vi "testAndMeasure.vi"() -> ()   [LabVIEW 2016]
uses:
  Anemometry/Anemometry Sub Vis/Controls/Post_Process.ctl
  Anemometry/Anemometry Sub Vis/Controls/Save_Data.ctl
  Anemometry/Anemometry Sub Vis/Controls/Setup.ctl
  Anemometry/Anemometry Sub Vis/Globals/Meas_global.vi
panel:
  in  "Measure (seconds)":dbl=10.0
  in  "Stop Button":bool
  in  "ResultsFilename":string="StaircaseTest"
  in  "settling(s)":u32=10
  out "conc":dbl=2.0 format="%.2f"
  out "flow":dbl=10.0 format="%.2f"
  in  "flowStep":dbl=10.0
  in  "flowMax":dbl=100.0
  in  "concMax":dbl=10.0
  in  "concStep":dbl=1.0
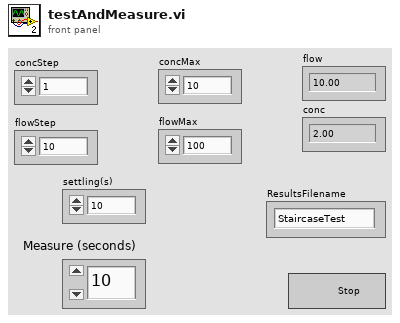
[diagram p1: front panel]
types:
  T1 = typedef "Setup.ctl" = enum16{"Run Program", "Show Setup", "Save Current Setup", "Setup Front Panel"}
  T2 = typedef "Save_Data.ctl" = enum16{"Save No Data", "Save Data"}
  T3 = typedef "Post_Process.ctl" = enum16{"Take New Data", "Post Process Raw Data File"}
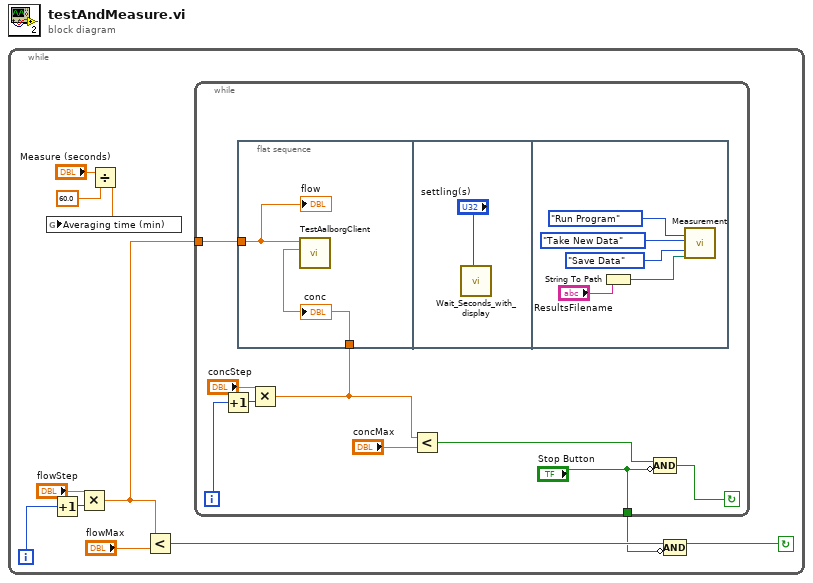
[diagram p0: block diagram]
diagram:
  n1 = while {
    i -> [w9]
    stop <- w2 continue-if-true
    n2 = Increment(x=w9) -> (x+1=w10:i32)
    n3 = Multiply(x="flowStep", y=w10) -> (x*y=w6:dbl)
    n4 = Divide(x="Measure (seconds)", y=60.0 ("x")) -> (x/y=w3:dbl)
    n5 = global write "Meas_global.vi" "Averaging time (min)"(w3) -> ()
    n6 = Less?(x=w6, y="flowMax") -> (x < y?=w8:bool)
    n7 = while {
      tunnel: w6 -> [w16]
      tunnel: ["Stop Button"] -> w1
      i -> [w20]
      stop <- w13 continue-if-true
      n8 = Increment(x=w20) -> (x+1=w19:i32)
      n9 = flat-sequence {
        tunnel: w16 -> [w22]
        tunnel: w15 -> [w21]
        frame #0 {
          n10 = call "TestAalborgClient.vi"("C_dem:(%)"=w21, "Q_dem[Total]:(l/min)"=w22) -> ()  [unwired: 10 in]
          "flow" <- w22
          "conc" <- w21
        }
        frame #1 {
          n11 = call "Wait_Seconds_with_display.vi"("Seconds to wait"="settling(s)") -> ()  [unwired: 2 in, 1 out]
        }
        frame #2 {
          n12 = String To Path(string="ResultsFilename") -> (path=w28:path)
          n13 = call "Measurement.vi"("setup"=Setup."Run Program", "Post Process"=Post_Process."Take New Data", "File"=Save_Data."Save Data", "Results file"=w28) -> ()  [unwired: 3 in, 13 out]
        }
      }
      n14 = Multiply(x="concStep", y=w19) -> (x*y=w15:dbl)
      n15 = Less?(x=w15, y="concMax") -> (x < y?=w14:bool)
      n16 = Compound Arithmetic op=AND(w14, invert "Stop Button") -> (w13:bool)
    }
    n17 = Compound Arithmetic op=AND(w8, invert w1) -> (w2:bool)
  }
